vi "Example_Local MQTT Communication.vi"() -> ()   [LabVIEW 2013]
uses:
  Control Packets/ControlPacket/Control Packet Type -- enum.ctl
  Control Packets/ControlPacket/ControlPacket.lvclass
  Control Packets/CONNACK/Connect Return Code -- enum.ctl
  Control Packets/SUBSCRIBE/Topic Subscription -- cluster.ctl
  Control Packets/ControlPacket/QualityOfService -- enum.ctl
  Control Packets/SUBACK/Subscription Success Code.ctl
  Control Packets/CONNECT/Create CONNECT Packet.vi
  Control Packets/CONNACK/Create CONNACK Packet.vi
  Control Packets/PINGRESP/Create PINGRESP Packet.vi
  Control Packets/DISCONNECT/Create DISCONNECT Packet.vi
  Control Packets/AUTH/Create AUTH Packet.vi
  Control Packets/PUBLISH/Create PUBLISH Packet (Server).vi
  Control Packets/PUBACK/Create PUBACK Packet.vi
  Control Packets/PUBREC/Create PUBREC Packet.vi
  Control Packets/PUBREL/Create PUBREL Packet.vi
  Control Packets/PUBCOMP/Create PUBCOMP Packet.vi
  Control Packets/SUBSCRIBE/Create SUBSCRIBE Packet.vi
  Control Packets/SUBACK/Create SUBACK Packet.vi
  Control Packets/UNSUBSCRIBE/Create UNSUBSCRIBE Packet.vi
  Control Packets/UNSUBACK/Create UNSUBACK Packet.vi
  Control Packets/CONNACK/CONNACK.lvclass
  Control Packets/PINGREQ/PINGREQ.lvclass
  Control Packets/PINGRESP/PINGRESP.lvclass
  Control Packets/PUBACK/PUBACK.lvclass
  Control Packets/UNSUBACK/UNSUBACK.lvclass
  Control Packets/UNSUBSCRIBE/UNSUBSCRIBE.lvclass
  Control Packets/SUBSCRIBE/SUBSCRIBE.lvclass
  Control Packets/SUBACK/SUBACK.lvclass
  Control Packets/MQTT_311/MQTTVersion.lvclass
  Control Packets/CONNECT/CONNECT.lvclass
  Control Packets/DISCONNECT/DISCONNECT.lvclass
  Control Packets/AUTH/AUTH.lvclass
  Control Packets/PUBLISH/PUBLISH.lvclass
  Control Packets/PUBREC/PUBREC.lvclass
  Control Packets/PUBREL/PUBREL.lvclass
  Control Packets/PUBCOMP/PUBCOMP.lvclass
panel:
  in  "Control Packet Type":T1
  in  "Send":bool
  out "Packets Received":T1[](array[typedef])
  # "This list indicates which packets were received by the client loop"
  # "^^\nPress this button to send\na new packet to the client loop"
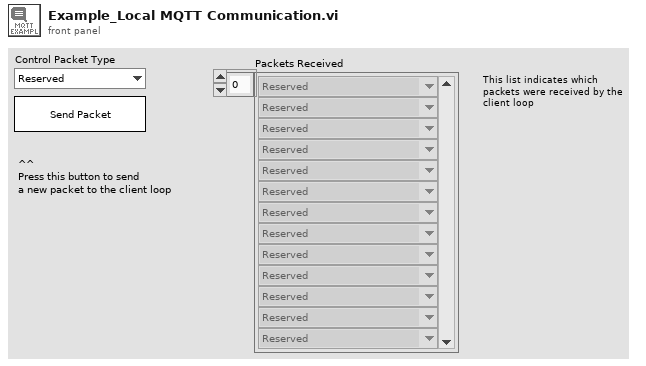
[diagram p1: front panel]
types:
  T1 = typedef "MQTT_Control_Packets.lvlib/ControlPacket.lvclass/Control Packet Type -- enum.ctl" = enum16{"Reserved", "CONNECT", "CONNACK", "PUBLISH", "PUBACK", "PUBREC", "PUBREL", "PUBCOMP", "SUBSCRIBE", "SUBACK", "UNSUBSCRIBE", "UNSUBACK", "PINGREQ", "PINGRESP", "DISCONNECT", "AUTH"}
  T2 = typedef "MQTT_Control_Packets.lvlib/CONNACK.lvclass/Connect Return Code -- enum.ctl" = enum16{"Connection accepted", "Unacceptable protocol version", "Identifier Rejected", "Server Unavailable", "Bad Username or Password", "Not Authorized"}
  T3 = typedef "MQTT_Control_Packets.lvlib/SUBSCRIBE.lvclass/Topic Subscription -- cluster.ctl" = cluster{"Topic Filter":string, "QoS":T4}
  T4 = typedef "MQTT_Control_Packets.lvlib/ControlPacket.lvclass/QualityOfService -- enum.ctl" = enum16{"0 (At Most Once)", "1 (At Least Once)", "2 (Exactly Once)"}
  T5 = typedef "MQTT_Control_Packets.lvlib/SUBACK.lvclass/Subscription Success Code.ctl" = cluster{"Subscription Failure":bool, "QoS":T4}
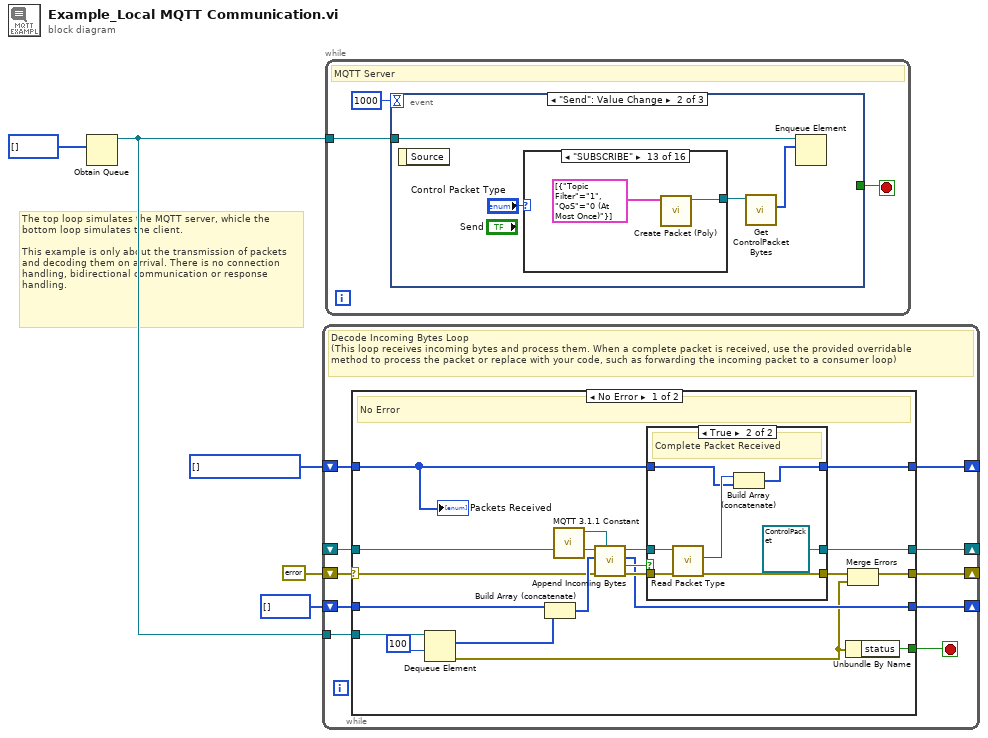
[diagram p0: block diagram]
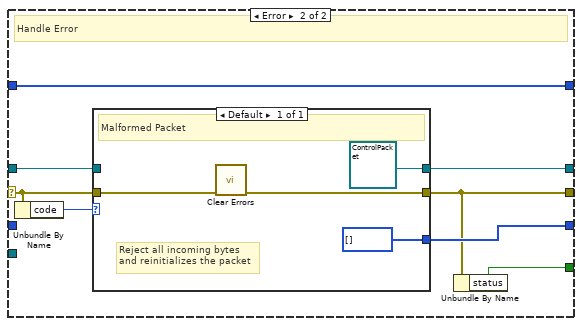
[diagram p3: hidden frame]
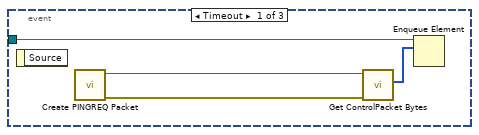
[diagram p4: hidden frame]
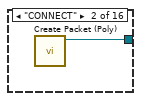
[diagram p6: hidden frame]
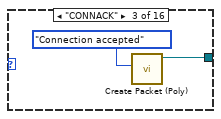
[diagram p7: hidden frame]
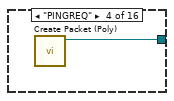
[diagram p8: hidden frame]
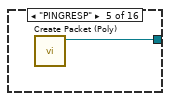
[diagram p9: hidden frame]
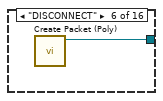
[diagram p10: hidden frame]
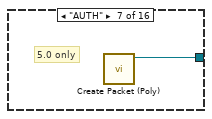
[diagram p11: hidden frame]
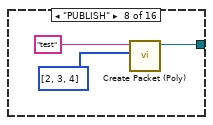
[diagram p12: hidden frame]
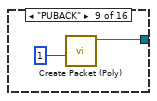
[diagram p13: hidden frame]
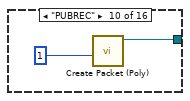
[diagram p14: hidden frame]
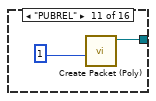
[diagram p15: hidden frame]
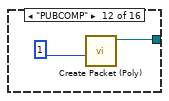
[diagram p16: hidden frame]
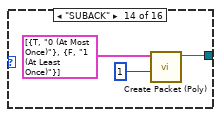
[diagram p17: hidden frame]
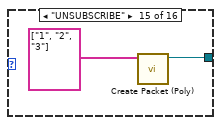
[diagram p18: hidden frame]
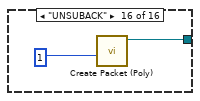
[diagram p19: hidden frame]
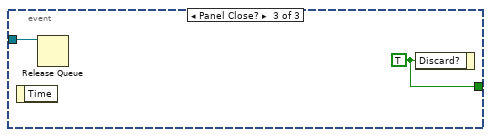
[diagram p20: hidden frame]
diagram:
  w1 = T1[] [] items=["Reserved", "CONNECT", "CONNACK", "PUBLISH", "PUBACK", "PUBREC", "PUBREL", "PUBCOMP", "SUBSCRIBE", "SUBACK", "UNSUBSCRIBE", "UNSUBACK", "PINGREQ", "PINGRESP", "DISCONNECT", "AUTH"]
  # "The top loop simulates the MQTT server, whicle the bottom loop simulates the client.\n\nThis example is only about the transmission of packets and decoding them on arrival. There is no connection handling, bidirectional communication or response handling."
  n1 = Obtain Queue(element data type=u8[] [] ("Remaining Packets")) -> (queue out=w2:refnum<queue>)  [unwired: 4 in, 2 out]
  n2 = while {
    shift-right: [w13] -> _
    shift-left: u8[] [] ("Remaining Packets") -> [w12]
    shift-right: [w11] -> _
    shift-left: errorcluster {"status"=FALSE, "code"=0, "source"=""} ("error out") -> [w10]
    shift-right: [w14] -> _
    shift-left: _ -> [w15]
    tunnel: w2 -> [w8]
    shift-right: [w6] -> _
    shift-left: w1 -> [w7]
    stop <- w9 stop-if-true
    # "Decode Incoming Bytes Loop\n(This loop receives incoming bytes and process them. When a complete packet is received, use the provided overridable \nmethod to process the packet or replace with your code, such as forwarding the incoming packet to a consumer loop)"
    n3 = case shown="No Error" w10 {
      selector: w10 -> [w23 w48]
      tunnel: w15 -> [w34 w46]
      tunnel: [w29 w50] -> w14
      tunnel: [w27 w49] -> w13
      tunnel: w12 -> [w26 _]
      tunnel: [w24 w45] -> w11
      tunnel: [w18 w44] -> w9
      tunnel: w8 -> [w22 _]
      tunnel: w7 -> [w17 w43]
      tunnel: [w16 w43] -> w6
      frame No Error {
        # "No Error"
        n4 = Dequeue Element(queue=w22, timeout in ms (-1)=100) -> (element=w20:u8[], error out=w19:errorcluster)  [unwired: 1 in, 2 out]
        n5 = Build Array (concatenate)(w26, w20) -> (w33:u8[])
        n6 = call "MQTT 3.1.1 Constant.vi"() -> ("MQTT 3.1.1"=w32:refnum<class "MQTTVersion.lvclass">)  [unwired: 11 in]
        n7 = call "Append Incoming Bytes.vi"("MQTT Version (3.1.1)"=w32, "error in (no error)"=w23, "Incoming Packets"=w33, "Incomplete ControlPacket"=w34) -> ("error out"=w28:errorcluster, "Complete Packet"=w31:bool, "Remaining Packets"=w27:u8[], "ControlPacket"=w30:refnum<class "ControlPacket.lvclass">)  [unwired: 4 in]
        n8 = case shown="True" w31 {
          tunnel: w30 -> [w36 w41]
          tunnel: [w36 refnum<class "ControlPacket.lvclass"> refnum ("ControlPacket")] -> w29
          tunnel: [_ w40] -> w25
          tunnel: w28 -> [_ w40]
          tunnel: w17 -> [w35 w38]
          tunnel: [w35 w37] -> w16
          frame False {
            # "None or Partial Packet received"
          }
          frame True {
            # "Complete Packet Received"
            n9 = call "Read Packet Type.vi"("ControlPacket in"=w41) -> ("Control Packet Type"=w39:T1)  [unwired: 9 in, 1 out]
            n10 = Build Array (concatenate)(w39, w38) -> (w37:T1[])
          }
        }
        n11 = Unbundle By Name(w19) -> ("status"=w18:bool)
        n12 = Merge Errors(w25, w19) -> (w24:errorcluster)
        "Packets Received" <- w17
      }
      frame Error {
        # "Handle Error"
        n13 = Unbundle By Name(w48) -> ("code"=w47:i32)
        n14 = case shown="Default" w47 {
          tunnel: [refnum<class "ControlPacket.lvclass"> refnum ("ControlPacket")] -> w50
          tunnel: w48 -> [w53]
          tunnel: [w52] -> w45
          tunnel: [u8[] [] ("Remaining Packets")] -> w49
          tunnel: w46 -> [_]
          frame Default {
            # "Reject all incoming bytes\nand reinitializes the packet"
            # "Malformed Packet"
            n15 = call <vilib>:"Clear Errors.vi"("error in (no error)"=w53) -> ("error out"=w52:errorcluster)  [unwired: 6 in]
          }
        }
        n16 = Unbundle By Name(w45) -> ("status"=w44:bool)
      }
    }
  }
  n17 = while {
    tunnel: w2 -> [w56]
    stop <- w55 stop-if-true
    # "MQTT Server"
    n18 = event shown="[1] \"Send\": Value Change" {
      selector: _ -> [_ _ _]
      dyn-events: _ -> [_ _ _]
      timeout: 1000 -> [_ _ _]
      tunnel: w56 -> [w61 w65 w93]
      tunnel: [_ _ w94] -> w55
      event Timeout {
        n19 = event-data() -> ()  [unwired: 1 in, 1 out]
        n20 = call "Create PINGREQ Packet.vi"() -> ("error out"=w60:errorcluster, "PINGREQ out"=w59:refnum<class "PINGREQ.lvclass">)  [unwired: 10 in]
        n21 = call "Get ControlPacket Bytes.vi"("error in (no error)"=w60, "ControlPacket"=w59) -> ("Bytes Stream"=w58:u8[])  [unwired: 6 in, 3 out]
        n22 = Enqueue Element(queue=w61, element=w58) -> ()  [unwired: 2 in, 3 out]
      }
      event "Send": Value Change {
        n23 = event-data() -> ()  [unwired: 1 in, 1 out]
        n24 = case shown="\"SUBSCRIBE\"" "Control Packet Type" {
          tunnel: [_ w66 w67 w69 w70 w71 w72 w75 w76 w79 w81 w83 w84 w87 w90 w92] -> w62
          frame "Reserved" {
          }
          frame "CONNECT" {
            n25 = call-poly "Create Packet (Poly).vi"() -> ("CONNECT"=w66:refnum<class "CONNECT.lvclass">)  [unwired: 10 in, 1 out]
          }
          frame "CONNACK" {
            n26 = call-poly "Create Packet (Poly).vi"("Return Code"=Connect_Return_Code_--_enum."Connection accepted") -> ("CONNACK"=w67:refnum<class "CONNACK.lvclass">)  [unwired: 9 in, 1 out]
          }
          frame "PINGREQ" {
            n27 = call-poly "Create Packet (Poly).vi"() -> ("PINGREQ out"=w69:refnum<class "PINGREQ.lvclass">)  [unwired: 10 in, 1 out]
          }
          frame "PINGRESP" {
            n28 = call-poly "Create Packet (Poly).vi"() -> ("PINGRESP out"=w70:refnum<class "PINGRESP.lvclass">)  [unwired: 10 in, 1 out]
          }
          frame "DISCONNECT" {
            n29 = call-poly "Create Packet (Poly).vi"() -> ("DISCONNECT"=w71:refnum<class "DISCONNECT.lvclass">)  [unwired: 10 in, 1 out]
          }
          frame "AUTH" {
            # "5.0 only"
            n30 = call-poly "Create Packet (Poly).vi"() -> ("AUTH"=w72:refnum<class "AUTH.lvclass">)  [unwired: 10 in, 1 out]
          }
          frame "PUBLISH" {
            n31 = call-poly "Create Packet (Poly).vi"("Payload"=u8[] [2, 3, 4], "Topic Name"="test") -> ("PUBLISH"=w75:refnum<class "PUBLISH.lvclass">)  [unwired: 7 in, 2 out]
          }
          frame "PUBACK" {
            n32 = call-poly "Create Packet (Poly).vi"("Packet ID"=u16 1) -> ("PUBACK out"=w76:refnum<class "PUBACK.lvclass">)  [unwired: 9 in, 1 out]
          }
          frame "PUBREC" {
            n33 = call-poly "Create Packet (Poly).vi"("Packet ID"=u16 1) -> ("PUBREC out"=w79:refnum<class "PUBREC.lvclass">)  [unwired: 9 in, 1 out]
          }
          frame "PUBREL" {
            n34 = call-poly "Create Packet (Poly).vi"("Packet ID"=u16 1) -> ("PUBREL out"=w81:refnum<class "PUBREL.lvclass">)  [unwired: 9 in, 1 out]
          }
          frame "PUBCOMP" {
            n35 = call-poly "Create Packet (Poly).vi"("Packet ID"=u16 1) -> ("PUBCOMP out"=w83:refnum<class "PUBCOMP.lvclass">)  [unwired: 9 in, 1 out]
          }
          frame "SUBSCRIBE" {
            n36 = call-poly "Create Packet (Poly).vi"("Topic Subscriptions"=T3[] [{"Topic Filter"="1", "QoS"=enum."0 (At Most Once)"}]) -> ("SUBSCRIBE out"=w84:refnum<class "SUBSCRIBE.lvclass">)  [unwired: 9 in, 1 out]
          }
          frame "SUBACK" {
            n37 = call-poly "Create Packet (Poly).vi"("Packet ID"=u16 1, "Return Codes"=T5[] [{"Subscription Failure"=TRUE, "QoS"=enum."0 (At Most Once)"}, {"Subscription Failure"=FALSE, "QoS"=enum."1 (At Least Once)"}]) -> ("SUBACK"=w87:refnum<class "SUBACK.lvclass">)  [unwired: 8 in, 1 out]
          }
          frame "UNSUBSCRIBE" {
            n38 = call-poly "Create Packet (Poly).vi"("Topic Subscriptions"=string[] ["1", "2", "3"]) -> ("UNSUBSCRIBE out"=w90:refnum<class "UNSUBSCRIBE.lvclass">)  [unwired: 9 in, 1 out]
          }
          frame "UNSUBACK" {
            n39 = call-poly "Create Packet (Poly).vi"("Packet ID"=u16 1) -> ("UNSUBACK out"=w92:refnum<class "UNSUBACK.lvclass">)  [unwired: 9 in, 1 out]
          }
        }
        n40 = call "Get ControlPacket Bytes.vi"("ControlPacket"=w62) -> ("Bytes Stream"=w64:u8[])  [unwired: 7 in, 3 out]
        n41 = Enqueue Element(queue=w65, element=w64) -> ()  [unwired: 2 in, 3 out]
      }
      event Panel Close? {
        w94 = TRUE ("Discard?")
        n42 = event-data() -> ()  [unwired: 1 in, 1 out]
        n43 = Release Queue(queue=w93) -> ()  [unwired: 2 in, 3 out]
        n44 = event-data("Discard?"=w94) -> ()  [unwired: 1 in, 1 out]
      }
    }
  }
